vi "ReadSystemParameters_SM.vi"(7 "error in (no error)":errorcluster, 9 "Override File Path":path=path "C:/Users/veenaj/Desktop/ZenGage V1.3/Configuration file/Zengage System JSON Override.json", 10 "Default File Path":path=path "E:/ZenGage V1.3.1/Configuration file/Zengage System Parameters.json") -> (0 "error out":errorcluster, 3 "System Parameters":T1)   [LabVIEW 2019, in "Inspection Statemachine.lvclass"]
uses:
  Inspection Statemachine.lvclass
panel:
  in  "Cluster":T2
  out "Error Message":string
  out "VCluster\n out":variant
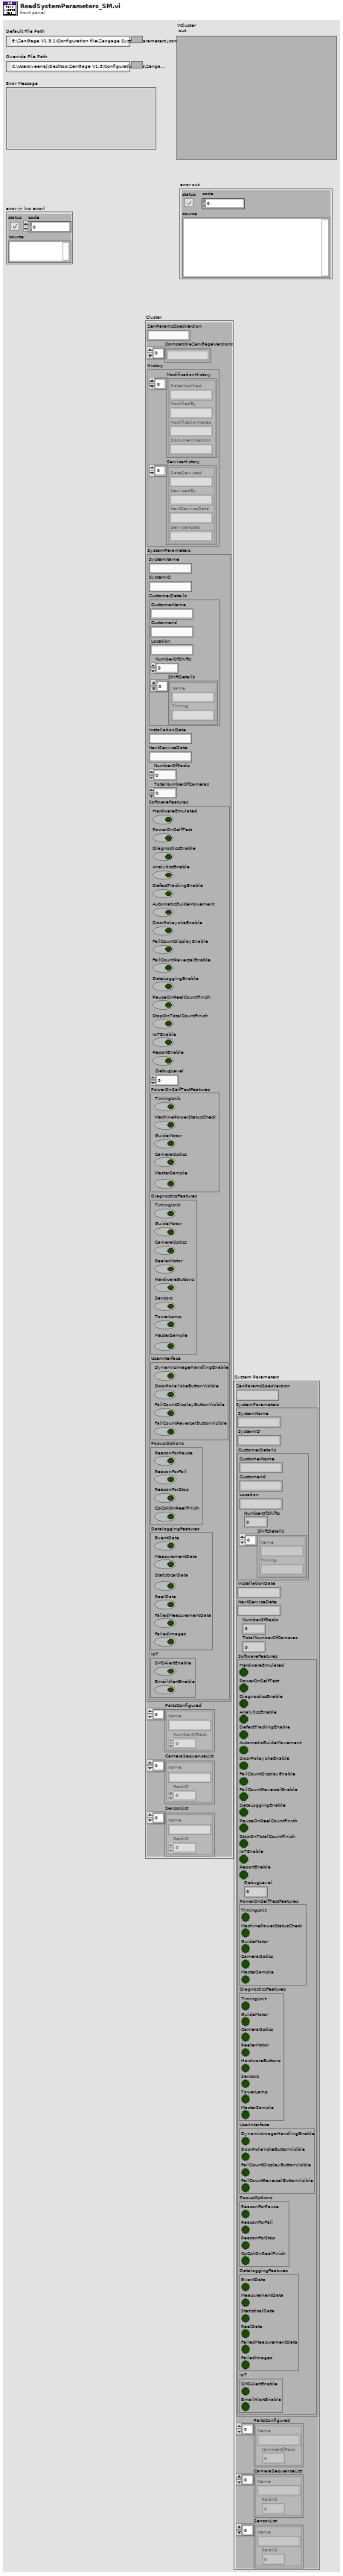
[diagram p1: front panel]
types:
  T1 = cluster{"ZenParamsSpecVersion":string, "SystemParameters":cluster{"SystemName":string, "SystemID":string, "CustomerDetails":cluster{"CustomerName":string, "CustomerId":string, "Location":string, "NumberOfShifts":dbl, "ShiftDetails":cluster{"Name":string, "Timing":string}[]}, "InstallationDate":string, "NextServiceDate":string, "NumberOfRacks":u8, "TotalNumberOfCameras":u8, "SoftwareFeatures":cluster{"HardwareEmulated":bool, "PowerOnSelfTest":bool, "DiagnosticsEnable":bool, "AnalyticsEnable":bool, "DefectTrackingEnable":bool, "AutomaticGuideMovement":bool, "DoorPokayokeEnable":bool, "FailCountDisplayEnable":bool, "FailCountReversalEnable":bool, "DataLoggingEnable":bool, "PauseOnReelCountFinish":bool, "StopOnTotalCountFinish":bool, "IoTEnable":bool, "ReportEnable":bool, "DebugLevel":dbl, "PowerOnSelfTestFeatures":cluster{"TimingUnit":bool, "MachinePowerStatusCheck":bool, "GuideMotor":bool, "CameraOptics":bool, "MasterSample":bool}, "DiagnosticsFeatures":cluster{"TimingUnit":bool, "GuideMotor":bool, "CameraOptics":bool, "ReelerMotor":bool, "HardwareButtons":bool, "Sensors":bool, "TowerLamp":bool, "MasterSample":bool}, "UserInterface":cluster{"DynamicImageHandlingEnable":bool, "DoorPokaYokeButtonVisible":bool, "FailCountDisplayButtonVisible":bool, "FailCountReversalButtonVisible":bool}, "PopupOptions":cluster{"ReasonForPause":bool, "ReasonForFail":bool, "ReasonForStop":bool, "CpCpkOnReelFinish":bool}, "DataloggingFeatures":cluster{"EventData":bool, "MeasurementData":bool, "StatisticalData":bool, "ReelData":bool, "FailedMeasurementData":bool, "FailedImages":bool}, "IoT":cluster{"SMSAlertEnable":bool, "EmailAlertEnable":bool}}}, "PartsConfigured":cluster{"Name":string, "NumberOfRack":u8}[], "CameraSequenceList":cluster{"Name":string, "RackID":u8}[], "SensorList":cluster{"Name":string, "RackID":u8}[]}
  T2 = cluster{"ZenParamsSpecVersion":string, "CompatibleZenGageVersions":string[], "History":cluster{"ModificationHistory":cluster{"DateModified":string, "ModifiedBy":string, "ModificationNotes":string, "DocumentVersion":string}[], "ServiceHistory":cluster{"DateServiced":string, "ServicedBy":string, "NextServiceDate":string, "ServiceNotes":string}[]}, "SystemParameters":cluster{"SystemName":string, "SystemID":string, "CustomerDetails":cluster{"CustomerName":string, "CustomerId":string, "Location":string, "NumberOfShifts":dbl, "ShiftDetails":cluster{"Name":string, "Timing":string}[]}, "InstallationDate":string, "NextServiceDate":string, "NumberOfRacks":u8, "TotalNumberOfCameras":u8, "SoftwareFeatures":cluster{"HardwareEmulated":bool, "PowerOnSelfTest":bool, "DiagnosticsEnable":bool, "AnalyticsEnable":bool, "DefectTrackingEnable":bool, "AutomaticGuideMovement":bool, "DoorPokayokeEnable":bool, "FailCountDisplayEnable":bool, "FailCountReversalEnable":bool, "DataLoggingEnable":bool, "PauseOnReelCountFinish":bool, "StopOnTotalCountFinish":bool, "IoTEnable":bool, "ReportEnable":bool, "DebugLevel":dbl, "PowerOnSelfTestFeatures":cluster{"TimingUnit":bool, "MachinePowerStatusCheck":bool, "GuideMotor":bool, "CameraOptics":bool, "MasterSample":bool}, "DiagnosticsFeatures":cluster{"TimingUnit":bool, "GuideMotor":bool, "CameraOptics":bool, "ReelerMotor":bool, "HardwareButtons":bool, "Sensors":bool, "TowerLamp":bool, "MasterSample":bool}, "UserInterface":cluster{"DynamicImageHandlingEnable":bool, "DoorPokaYokeButtonVisible":bool, "FailCountDisplayButtonVisible":bool, "FailCountReversalButtonVisible":bool}, "PopupOptions":cluster{"ReasonForPause":bool, "ReasonForFail":bool, "ReasonForStop":bool, "CpCpkOnReelFinish":bool}, "DataloggingFeatures":cluster{"EventData":bool, "MeasurementData":bool, "StatisticalData":bool, "ReelData":bool, "FailedMeasurementData":bool, "FailedImages":bool}, "IoT":cluster{"SMSAlertEnable":bool, "EmailAlertEnable":bool}}}, "PartsConfigured":cluster{"Name":string, "NumberOfRack":u8}[], "CameraSequenceList":cluster{"Name":string, "RackID":u8}[], "SensorList":cluster{"Name":string, "RackID":u8}[]}
  T3 = cluster{"SystemName":string, "SystemID":string, "CustomerDetails":cluster{"CustomerName":string, "CustomerId":string, "Location":string, "NumberOfShifts":dbl, "ShiftDetails":cluster{"Name":string, "Timing":string}[]}, "InstallationDate":string, "NextServiceDate":string, "NumberOfRacks":u8, "TotalNumberOfCameras":u8, "SoftwareFeatures":cluster{"HardwareEmulated":bool, "PowerOnSelfTest":bool, "DiagnosticsEnable":bool, "AnalyticsEnable":bool, "DefectTrackingEnable":bool, "AutomaticGuideMovement":bool, "DoorPokayokeEnable":bool, "FailCountDisplayEnable":bool, "FailCountReversalEnable":bool, "DataLoggingEnable":bool, "PauseOnReelCountFinish":bool, "StopOnTotalCountFinish":bool, "IoTEnable":bool, "ReportEnable":bool, "DebugLevel":dbl, "PowerOnSelfTestFeatures":cluster{"TimingUnit":bool, "MachinePowerStatusCheck":bool, "GuideMotor":bool, "CameraOptics":bool, "MasterSample":bool}, "DiagnosticsFeatures":cluster{"TimingUnit":bool, "GuideMotor":bool, "CameraOptics":bool, "ReelerMotor":bool, "HardwareButtons":bool, "Sensors":bool, "TowerLamp":bool, "MasterSample":bool}, "UserInterface":cluster{"DynamicImageHandlingEnable":bool, "DoorPokaYokeButtonVisible":bool, "FailCountDisplayButtonVisible":bool, "FailCountReversalButtonVisible":bool}, "PopupOptions":cluster{"ReasonForPause":bool, "ReasonForFail":bool, "ReasonForStop":bool, "CpCpkOnReelFinish":bool}, "DataloggingFeatures":cluster{"EventData":bool, "MeasurementData":bool, "StatisticalData":bool, "ReelData":bool, "FailedMeasurementData":bool, "FailedImages":bool}, "IoT":cluster{"SMSAlertEnable":bool, "EmailAlertEnable":bool}}}
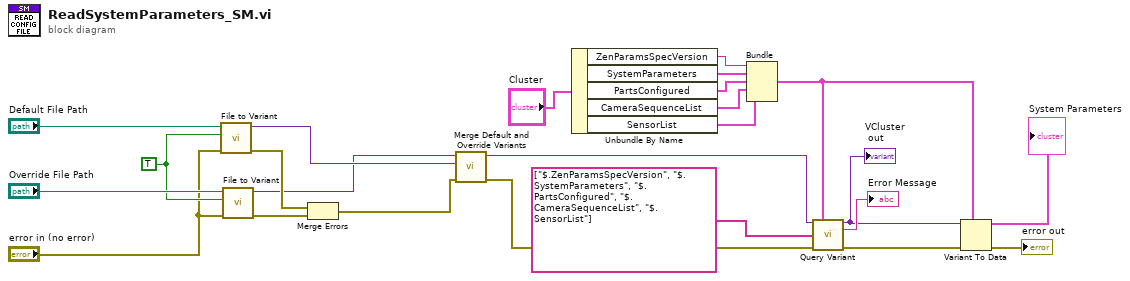
[diagram p0: block diagram]
diagram:
  w22 = TRUE ("Remove Comments?")
  n1 = call <vilib>:"File to Variant.vi"("JSON FilePath"="Default File Path", "Remove Comments?"=w22, "error in (no error)"="error in (no error)") -> ("JSON Variant"=w10:variant, "error out"=w20:errorcluster)  [unwired: 5 in, 1 out]
  n2 = call <vilib>:"File to Variant.vi"("JSON FilePath"="Override File Path", "Remove Comments?"=w22, "error in (no error)"="error in (no error)") -> ("JSON Variant"=w9:variant, "error out"=w19:errorcluster)  [unwired: 5 in, 1 out]
  n3 = Merge Errors(w20, w19) -> (w15:errorcluster)
  n4 = call <vilib>:"Merge Default and Override Variants.vi"("error in (no error)"=w15, "Default VCluster"=w10, "Override VCluster"=w9) -> ("error out"=w17:errorcluster, "Output Merged Cluster"=w14:variant)  [unwired: 7 in]
  n5 = Unbundle By Name("Cluster") -> ("ZenParamsSpecVersion"=w8:string, "SystemParameters"=w12:T3, "PartsConfigured"=w11:cluster{"Name":string, "NumberOfRack":u8}[], "CameraSequenceList"=w3:cluster{"Name":string, "RackID":u8}[], "SensorList"=w2:cluster{"Name":string, "RackID":u8}[])
  n6 = Bundle("ZenParamsSpecVersion"=w8, "SystemParameters"=w12, "PartsConfigured"=w11, "CameraSequenceList"=w3, "SensorList"=w2) -> (w4:T1)  [unwired: 1 in]
  n7 = call <vilib>:"Query Variant.vi"("VCluster in"=w14, "Reference Variant"=w4, "pathList"=string[] ["$.ZenParamsSpecVersion", "$.SystemParameters", "$.PartsConfigured", "$.CameraSequenceList", "$.SensorList"], "error IO"=w17) -> ("VCluster\n out"=w5:variant, "Error Message"=→"Error Message":string, "error out"=w7:errorcluster)  [unwired: 8 in, 1 out]
  "VCluster\n out" <- w5
  n8 = Variant To Data(error in=w7, type=w4, Variant=w5) -> (data=→"System Parameters":T1, error out=→"error out":errorcluster)
